vi "tcsWEP_logEvent_simParamList.vi"(8 "error in (no error)":errorcluster, 11 "logevent_simParamList_Ctl":T1) -> (0 "error out":errorcluster, 2 "function return":i32, 3 "logevent_simParamList_Ctl out":T1)   [LabVIEW 2016, in "SALLV_tcsWEP.lvlib"]
doc: "int tcsWEP_shm_logEvent_simParamListLV(tcsWEP_logevent_simParamListLV *logevent_simParamList_Ctl );"
uses:
  SALLV_tcsWEP.lvlib
  DataTypes/logevent_simParamList.ctl
  SALLV_tcsWEP.so
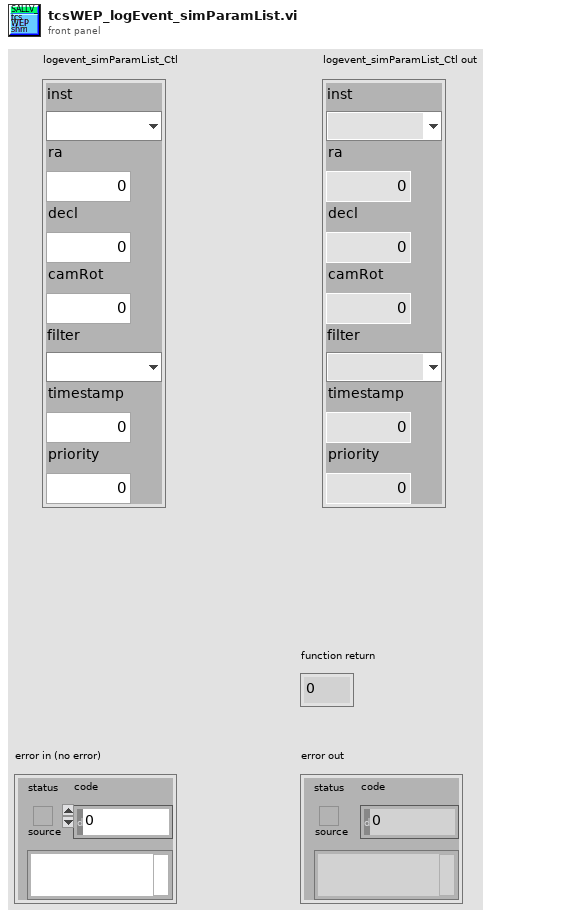
[diagram p1: front panel]
types:
  T1 = typedef "SALLV_tcsWEP.lvlib/logevent_simParamList.ctl" = cluster{"inst":enum32{"", "ComCam", "Lsst"}, "ra":i16, "decl":i16, "camRot":dbl, "filter":enum32{"", "Reference", "U", "G", "R", "I", "Z", "Y"}, "timestamp":dbl, "priority":i32}
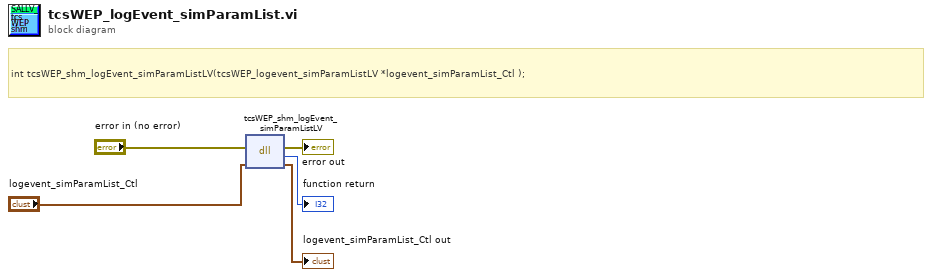
[diagram p0: block diagram]
diagram:
  # "int tcsWEP_shm_logEvent_simParamListLV(tcsWEP_logevent_simParamListLV *logevent_simParamList_Ctl );"
  n1 = dll-call lib="home/ttsai/Documents/salAPI/SALLV_tcsWEP.*" fn="tcsWEP_shm_logEvent_simParamListLV"(error in="error in (no error)", "logevent_simParamList_Ctl"="logevent_simParamList_Ctl") -> (error out=→"error out":errorcluster, →"function return":i32, "logevent_simParamList_Ctl"=→"logevent_simParamList_Ctl out":T1)  [unwired: 2 in, 1 out]
